vi "循环扫描脚本.vi"(8 "4-wire":bool, 9 "强制时序":bool, 11 "扫描":T1 {"NPLC" min=0.001 max=25.0 step=0.001; "- Δ V" min=0.0 max=1.0 format="%#_6pV"; "+ Δ V" min=0.0 max=1.0 format="%#_6pV"; "- V" min=-40.0 max=40.0 format="%#_6pV"; "- limit I" min=1e-08 max=3.0 format="%#_6pA"; "ΔT" format="%#_6ps"; "+ limit I" min=1e-08 max=3.0 format="%#_6pA"; "+ V" min=-40.0 max=40.0 format="%#_6pV"}) -> (3 "Script":string)   [LabVIEW 2020, in "功能选择.xctl"]
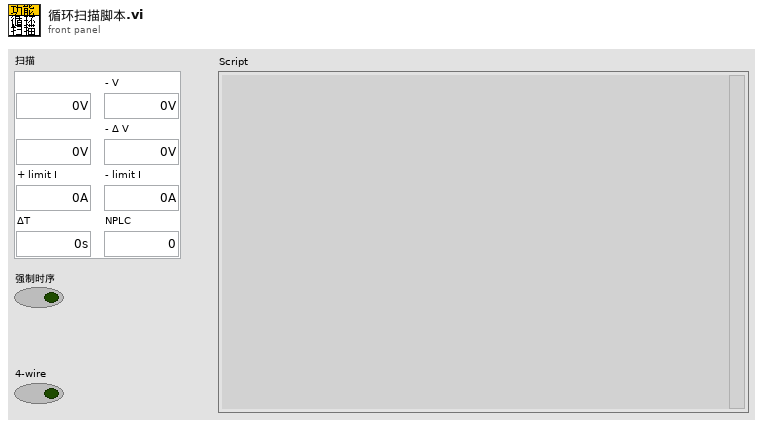
[diagram p1: front panel]
types:
  T1 = typedef "功能选择.xctl/扫描参数.ctl" = cluster{"+ V":dbl, "+ Δ V":dbl, "+ limit I":dbl, "- V":dbl, "- Δ V":dbl, "- limit I":dbl, "ΔT":dbl, "NPLC":dbl}
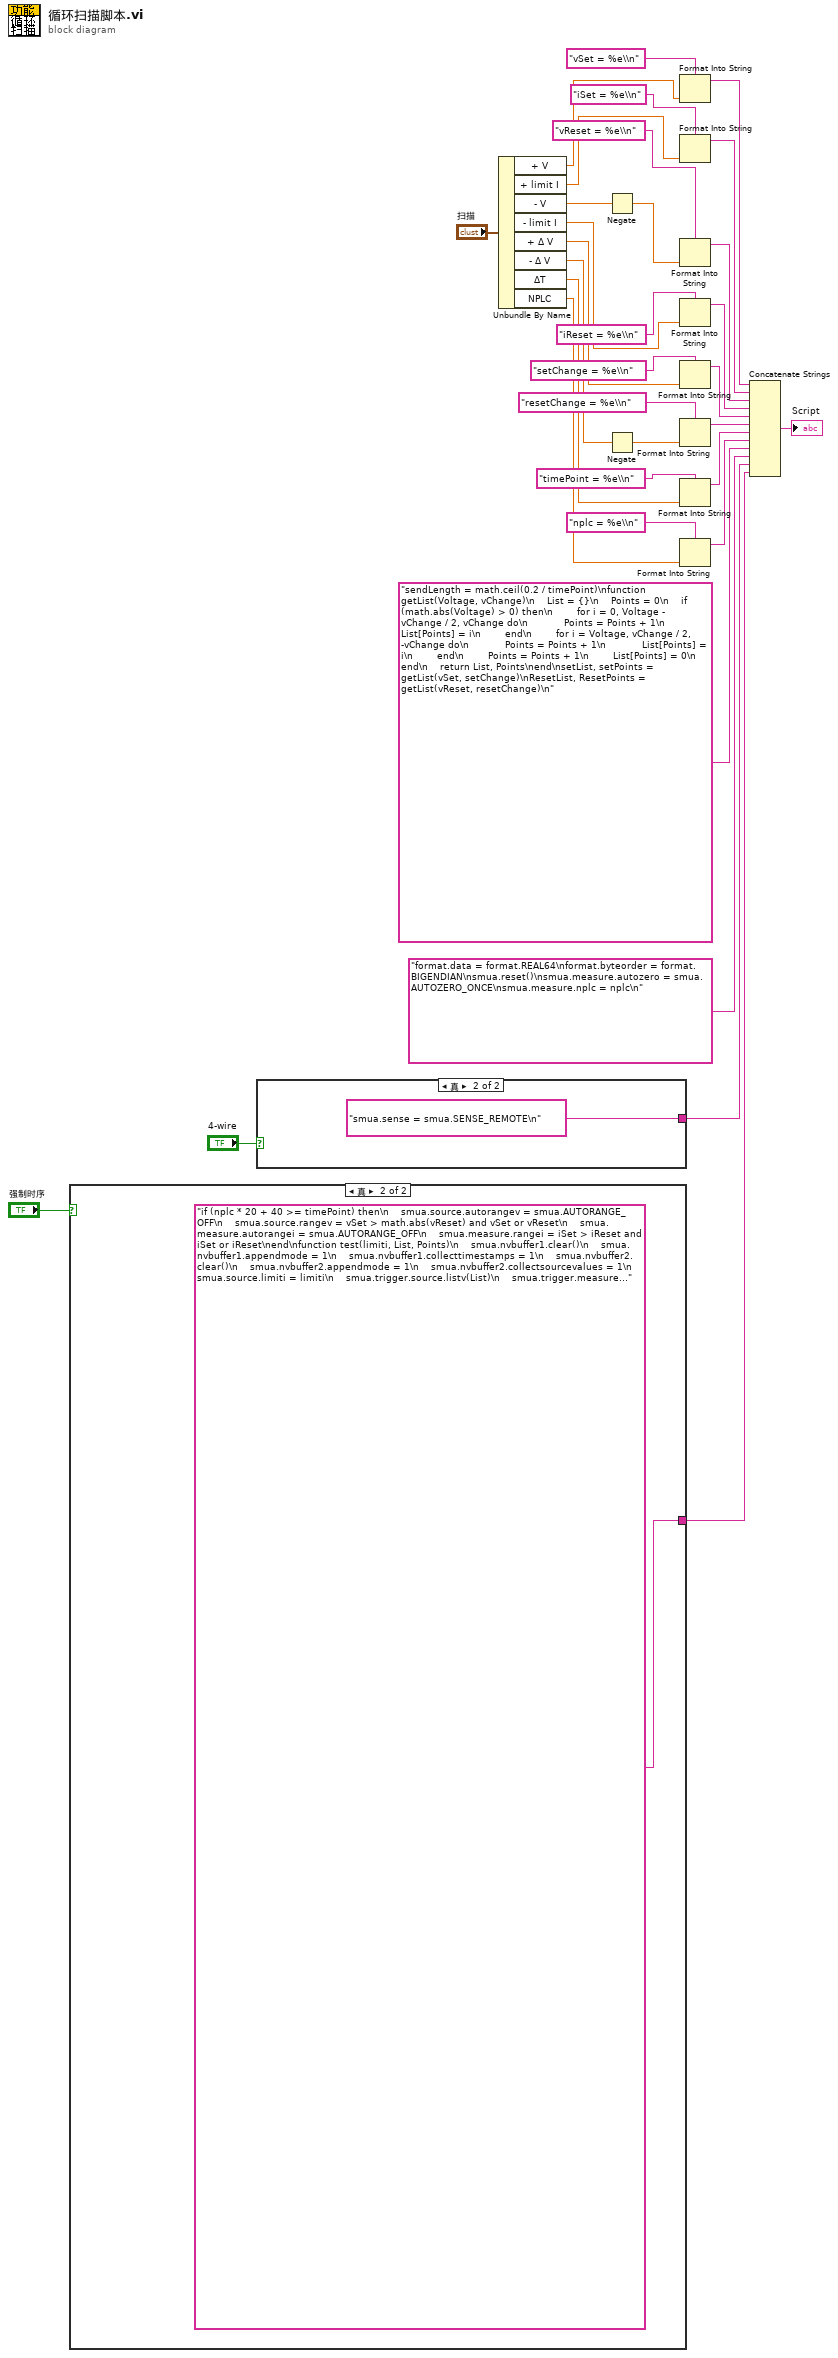
[diagram p0: block diagram]
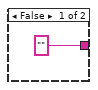
[diagram p2: hidden frame]
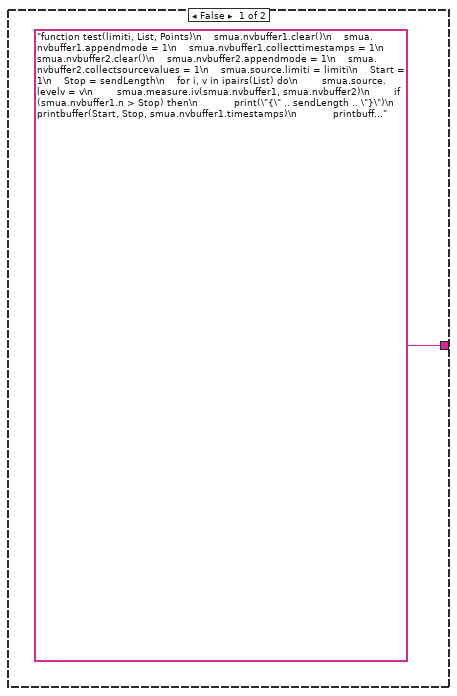
[diagram p3: hidden frame]
diagram:
  n1 = case shown="真" "强制时序" {
    tunnel: ["function test(limiti, List, Points)\n    smua.nvbuffer1.clear()\n    smua.nvbuffer1.appendmode = 1\n    smua.nvbuffer1.collecttimestamps = 1\n    smua.nvbuffer2.clear()\n    smua.nvbuffer2.appendmode = 1\n    smua.nvbuffer2.collectsourcevalues = 1\n    smua.source.limiti = limiti\n    Start = 1\n    Stop = sendLength\n    for i, v in ipairs(List) do\n        smua.source.levelv = v\n        smua.measure.iv(smua.nvbuffer1, smua.nvbuffer2)\n        if (smua.nvbuffer1.n > Stop) then\n            print(\"{\" .. sendLength .. \"}\")\n            printbuffer(Start, Stop, smua.nvbuffer1.timestamps)\n            printbuffer(Start, Stop, smua.nvbuffer2.sourcevalues)\n            printbuffer(Start, Stop, smua.nvbuffer1)\n            printbuffer(Start, Stop, smua.nvbuffer2)\n            Start = Start + sendLength\n            Stop = Stop + sendLength\n        end\n    end\n    Stop = Points\n    print(\"{\" .. Stop - Start + 1 .. \"}\")\n    printbuffer(Start, Stop, smua.nvbuffer1.timestamps)\n    printbuffer(Start, Stop, smua.nvbuffer2.sourcevalues)\n    printbuffer(Start, Stop, smua.nvbuffer1)\n    printbuffer(Start, Stop, smua.nvbuffer2)\n    print(\"{done}\")\nend\nsmua.source.output = smua.OUTPUT_ON\nif (setPoints > 0) then test(iSet, setList, setPoints) end\nif (ResetPoints > 0) then test(iReset, ResetList, ResetPoints) end\nsmua.source.output = smua.OUTPUT_OFF\nreset()\n" "if (nplc * 20 + 40 >= timePoint) then\n    smua.source.autorangev = smua.AUTORANGE_OFF\n    smua.source.rangev = vSet > math.abs(vReset) and vSet or vReset\n    smua.measure.autorangei = smua.AUTORANGE_OFF\n    smua.measure.rangei = iSet > iReset and iSet or iReset\nend\nfunction test(limiti, List, Points)\n    smua.nvbuffer1.clear()\n    smua.nvbuffer1.appendmode = 1\n    smua.nvbuffer1.collecttimestamps = 1\n    smua.nvbuffer2.clear()\n    smua.nvbuffer2.appendmode = 1\n    smua.nvbuffer2.collectsourcevalues = 1\n    smua.source.limiti = limiti\n    smua.trigger.source.listv(List)\n    smua.trigger.measure.iv(smua.nvbuffer1, smua.nvbuffer2)\n    smua.trigger.source.stimulus = trigger.timer[1].EVENT_ID\n    smua.trigger.source.action = smua.ENABLE\n    smua.trigger.measure.action = smua.ENABLE\n    smua.trigger.count = Points\n    smua.trigger.arm.stimulus = trigger.EVENT_ID\n    trigger.timer[1].reset()\n    trigger.timer[1].stimulus = smua.trigger.ARMED_EVENT_ID\n    trigger.timer[1].passthrough = false\n    trigger.timer[1].delay = timePoint\n    trigger.timer[1].count = Points\n    smua.trigger.initiate()\n    smua.trigger.arm.set()\nend\nfunction sendData()\n    Start = 1\n    Stop = sendLength\n    repeat\n        if (bit.test(status.operation.instrument.smua.condition, 4) == false) then\n            break\n        elseif (smua.nvbuffer1.n > Stop) then\n            print(\"{\" .. sendLength .. \"}\")\n            printbuffer(Start, Stop, smua.nvbuffer1.timestamps)\n            printbuffer(Start, Stop, smua.nvbuffer2.sourcevalues)\n            printbuffer(Start, Stop, smua.nvbuffer1)\n            printbuffer(Start, Stop, smua.nvbuffer2)\n            Start = Start + sendLength\n            Stop = Stop + sendLength\n        end\n        delay(timePoint)\n    until (false)\n    Stop = smua.nvbuffer1.n\n    print(\"{\" .. Stop - Start + 1 .. \"}\")\n    printbuffer(Start, Stop, smua.nvbuffer1.timestamps)\n    printbuffer(Start, Stop, smua.nvbuffer2.sourcevalues)\n    printbuffer(Start, Stop, smua.nvbuffer1)\n    printbuffer(Start, Stop, smua.nvbuffer2)\n    print(\"{done}\")\nend\nsmua.source.output = smua.OUTPUT_ON\nif (setPoints > 0) then\n    test(iSet, setList, setPoints)\n    sendData()\nend\nif (ResetPoints > 0) then\n    test(iReset, ResetList, ResetPoints)\n    sendData()\nend\nsmua.source.output = smua.OUTPUT_OFF\nreset()\n"] -> w26
    frame False {
    }
    frame True {
    }
  }
  n2 = case shown="真" "4-wire" {
    tunnel: ["" "smua.sense = smua.SENSE_REMOTE\n"] -> w25
    frame False {
    }
    frame True {
    }
  }
  n3 = Unbundle By Name("扫描") -> ("+ V"=w11:dbl, "+ limit I"=w10:dbl, "- V"=w9:dbl, "- limit I"=w8:dbl, "+ Δ V"=w7:dbl, "- Δ V"=w4:dbl, "ΔT"=w16:dbl, "NPLC"=w17:dbl)
  n4 = Negate(x=w9) -> (-x=w6:dbl)
  n5 = Negate(x=w4) -> (-x=w2:dbl)
  n6 = Format Into String(format string="vSet = %e\\n" ("格式字符串"), w11) -> (resulting string=w13:string)  [unwired: 2 in, 1 out]
  n7 = Format Into String(format string="iSet = %e\\n" ("格式字符串"), w10) -> (resulting string=w12:string)  [unwired: 2 in, 1 out]
  n8 = Format Into String(format string="vReset = %e\\n" ("格式字符串"), w6) -> (resulting string=w31:string)  [unwired: 2 in, 1 out]
  n9 = Format Into String(format string="iReset = %e\\n" ("格式字符串"), w8) -> (resulting string=w21:string)  [unwired: 2 in, 1 out]
  n10 = Format Into String(format string="setChange = %e\\n" ("格式字符串"), w7) -> (resulting string=w22:string)  [unwired: 2 in, 1 out]
  n11 = Format Into String(format string="resetChange = %e\\n" ("格式字符串"), w2) -> (resulting string=w3:string)  [unwired: 2 in, 1 out]
  n12 = Format Into String(format string="timePoint = %e\\n", w16) -> (resulting string=w20:string)  [unwired: 2 in, 1 out]
  n13 = Format Into String(format string="nplc = %e\\n", w17) -> (resulting string=w19:string)  [unwired: 2 in, 1 out]
  n14 = Concatenate Strings(w13, w12, w31, w21, w22, w3, w20, w19, "sendLength = math.ceil(0.2 / timePoint)\nfunction getList(Voltage, vChange)\n    List = {}\n    Points = 0\n    if (math.abs(Voltage) > 0) then\n        for i = 0, Voltage - vChange / 2, vChange do\n            Points = Points + 1\n            List[Points] = i\n        end\n        for i = Voltage, vChange / 2, -vChange do\n            Points = Points + 1\n            List[Points] = i\n        end\n        Points = Points + 1\n        List[Points] = 0\n    end\n    return List, Points\nend\nsetList, setPoints = getList(vSet, setChange)\nResetList, ResetPoints = getList(vReset, resetChange)\n", "format.data = format.REAL64\nformat.byteorder = format.BIGENDIAN\nsmua.reset()\nsmua.measure.autozero = smua.AUTOZERO_ONCE\nsmua.measure.nplc = nplc\n", w25, w26) -> (→"Script":string)
